vi "SLSC Dynamic Channel Lookups.vi"(6 "SLSCChannelPath":string="SLSCChannelPath", 8 "error in (no error)":errorcluster, 11 "Child Refs":T1[](array[typedef]) format="%.0x") -> (0 "error out":errorcluster, 3 "SLSC Dynamic Inputs":T2[](array[typedef]))   [LabVIEW 2017, in "SLSC EDS System Explorer.lvlib"]
uses:
  SLSC EDS System Explorer.lvlib
  SLSC CD API/SLSC CD Engine/SLSC Dynamic Channel.ctl
  SLSC CD API/SLSC CD Engine/SLSC Datatype.ctl
  <vilib>/NI Veristand/Custom Device API/Custom Device Item Ref.ctl
  <vilib>/NI Veristand/Custom Device API/Get Item Property (String).vi
  <vilib>/NI VeriStand/Custom Device API/Custom Device API.lvlib
  <vilib>/regexp/Match Regular Expression.xnode
  SLSC CD API/SLSC CD Shared/SLSC CD Shared.lvlib
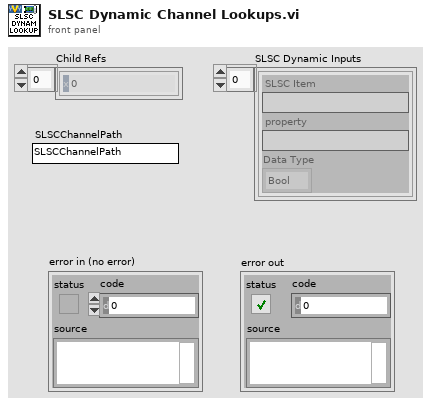
[diagram p1: front panel]
types:
  T1 = typedef "Custom Device API.lvlib/Custom Device Item Ref.ctl" = u64
  T2 = typedef "SLSC CD Shared.lvlib/SLSC Dynamic Channel.ctl" = cluster{"SLSC Item":string, "property":string, "Data Type":T3}
  T3 = typedef "SLSC CD Shared.lvlib/SLSC Datatype.ctl" = enum16{"Bool", "Double", "I32", "I64", "String", "U32", "U64"}
  T4 = enum16{"Bool", "Double", "I32", "I64", "String", "U32", "U64"}
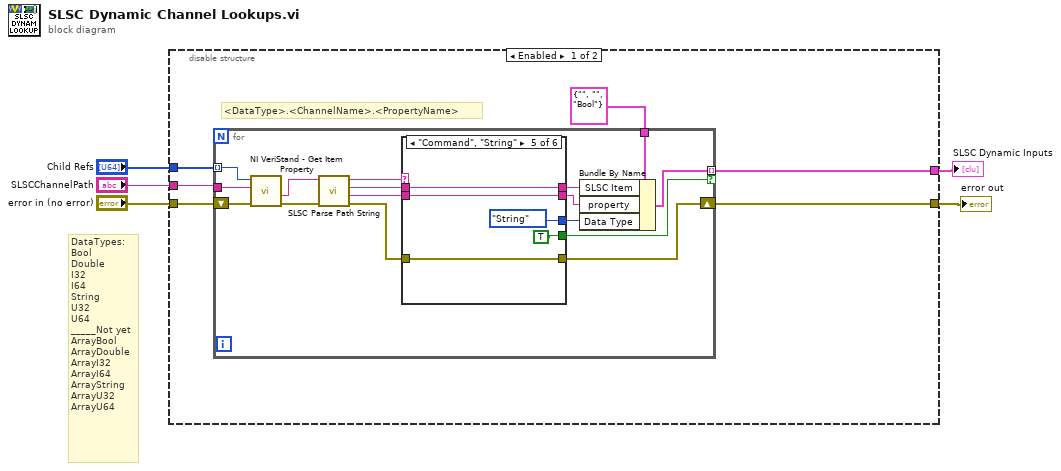
[diagram p0: block diagram]
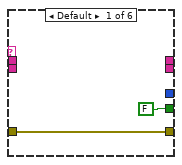
[diagram p2: hidden frame]
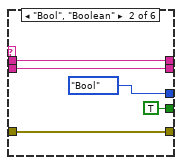
[diagram p3: hidden frame]
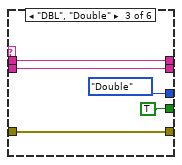
[diagram p4: hidden frame]
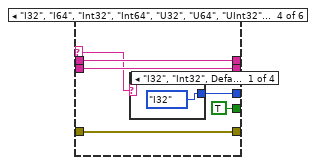
[diagram p5: hidden frame]
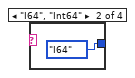
[diagram p6: hidden frame]
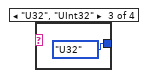
[diagram p7: hidden frame]
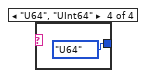
[diagram p8: hidden frame]
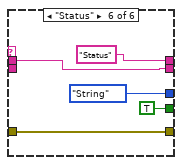
[diagram p9: hidden frame]
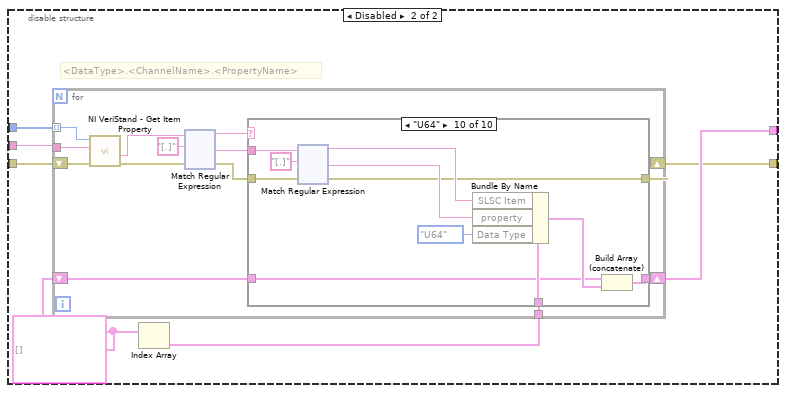
[diagram p10: hidden frame]
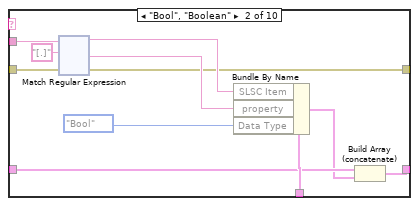
[diagram p12: hidden frame]
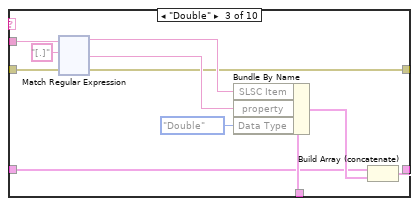
[diagram p13: hidden frame]
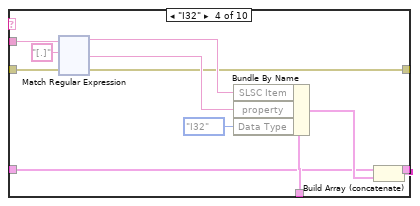
[diagram p14: hidden frame]
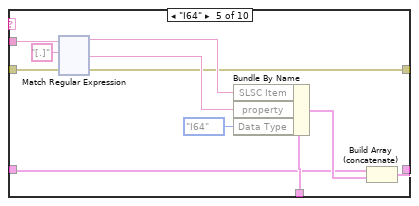
[diagram p15: hidden frame]
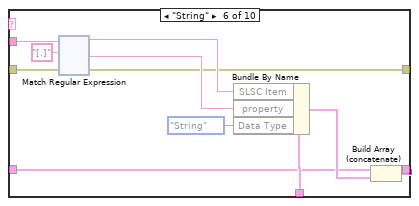
[diagram p16: hidden frame]
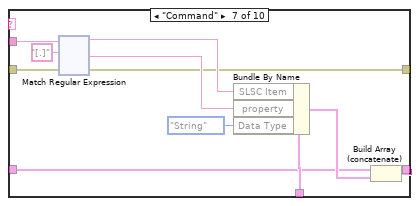
[diagram p17: hidden frame]
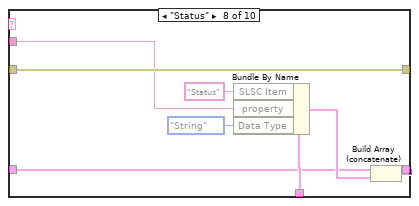
[diagram p18: hidden frame]
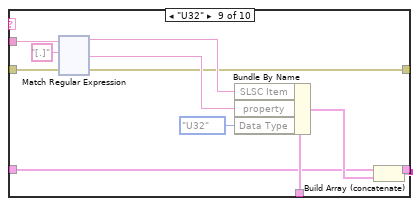
[diagram p19: hidden frame]
diagram:
  # "DataTypes:\nBool\nDouble\nI32\nI64\nString\nU32\nU64\n_____Not yet\nArrayBool\nArrayDouble\nArrayI32\nArrayI64\nArrayString\nArrayU32\nArrayU64"
  n1 = disable-structure shown="Enabled" {
    disable-tunnel: "Child Refs" -> [w11 w66]
    disable-tunnel: "error in (no error)" -> [w10 w65]
    disable-tunnel: [w7 w64] -> w3
    disable-tunnel: [w9 w63] -> w2
    disable-tunnel: "SLSCChannelPath" -> [w8 w62]
    frame Enabled {
      # "<DataType>.<ChannelName>.<PropertyName>"
      n2 = for {
        tunnel: w11 -> [w27] mode=indexing
        tunnel: w8 -> [w26]
        shift-right: [w24] -> w9
        shift-left: w10 -> [w25]
        tunnel: [w21] -> w7 mode=indexing if=w13
        tunnel: T2 {"SLSC Item"="", "property"="", "Data Type"=enum."Bool"} ("SLSC Dynamic Channel") -> [w12]
        n3 = call-poly <vilib>:"NI VeriStand - Get Item Property.vi"("error in (no error)"=w25, "Property Name"=w26, "Item Ref in"=w27) -> ("error out"=w15:errorcluster, "Value"=w23:string)  [unwired: 5 in, 2 out]
        n4 = call "SLSC Parse Path String.vi"("error in (no error)"=w15, "SLSC Channel Path"=w23) -> ("error out"=w14:errorcluster, "Property or Command"=w17:string, "Physical Channel"=w19:string, "Datatype"=w22:string)  [unwired: 6 in]
        n5 = case shown="\"Command\", \"String\"" w22 {
          selector: w22 -> [_ _ _ w41 _ _]
          tunnel: w14 -> [w29 w31 w36 w43 w51 w58]
          tunnel: [w29 w31 w36 w43 w51 w58] -> w24
          tunnel: [_ w34 w39 w45 w54 "Status" ("Physical Channel")] -> w20
          tunnel: w19 -> [_ w34 w39 w45 w54 w55]
          tunnel: [_ w33 w38 w44 w53 w55] -> w18
          tunnel: w17 -> [_ w33 w38 w44 w53 _]
          tunnel: [_ SLSC_Datatype."Bool" ("Data Type") SLSC_Datatype."Double" ("Data Type") w40 SLSC_Datatype."String" ("Data Type") SLSC_Datatype."String" ("Data Type")] -> w16
          tunnel: [FALSE TRUE TRUE TRUE TRUE TRUE] -> w13
          frame Default {
          }
          frame "Bool", "Boolean" {
          }
          frame "DBL", "Double" {
          }
          frame "I32", "I64", "Int32", "Int64", "U32", "U64", "UInt32", "UInt64" {
            n6 = case shown="\"I32\", \"Int32\", Default" w41 {
              tunnel: [SLSC_Datatype."I32" ("Data Type") SLSC_Datatype."I64" ("Data Type") SLSC_Datatype."U32" ("Data Type") SLSC_Datatype."U64" ("Data Type")] -> w40
              frame "I32", "Int32", Default {
              }
              frame "I64", "Int64" {
              }
              frame "U32", "UInt32" {
              }
              frame "U64", "UInt64" {
              }
            }
          }
          frame "Command", "String" {
          }
          frame "Status" {
          }
        }
        n7 = Bundle By Name(cluster=w12, "SLSC Item"=w20, "property"=w18, "Data Type"=w16) -> (w21:T2)
      }
    }
    frame Disabled {
      w60 = T2[] [] ("SLSC Dynamic Inputs")
      # "<DataType>.<ChannelName>.<PropertyName>"
      n8 = Index Array(array=w60) -> (element=w61:T2)  [unwired: 1 in]
      n9 = for {
        tunnel: w66 -> [w79] mode=indexing
        tunnel: w62 -> [w78]
        shift-right: [w67] -> w63
        shift-left: w65 -> [w73]
        tunnel: w61 -> [w70]
        shift-right: [w68] -> w64
        shift-left: w60 -> [w69]
        n10 = call-poly <vilib>:"NI VeriStand - Get Item Property.vi"("error in (no error)"=w73, "Property Name"=w78, "Item Ref in"=w79) -> ("error out"=w71:errorcluster, "Value"=w72:string)  [unwired: 5 in, 2 out]
        n11 = xnode "Match Regular Expression"("input string"=w72, "regular expression"="[.]", "error in"=w71) -> ("before match"=w75:string, "after match"=w76:string, "error out"=w77:errorcluster)  [unwired: 3 in, 2 out]
        n12 = case shown="\"U64\"" w75 {
          tunnel: w76 -> [_ w91 w216 w341 w466 w591 w716 w833 w849 w974]
          tunnel: w77 -> [w81 w90 w215 w340 w465 w590 w715 w834 w848 w973]
          tunnel: w70 -> [_ w87 w210 w337 w462 w587 w712 w839 w845 w970]
          tunnel: w69 -> [w80 w86 w208 w334 w458 w584 w709 w836 w841 w966]
          tunnel: [w80 w85 w211 w333 w459 w583 w708 w835 w843 w967] -> w68
          tunnel: [w81 w83 w207 w332 w457 w582 w707 w834 w840 w965] -> w67
          frame Default {
          }
          frame "Bool", "Boolean" {
            n13 = xnode "Match Regular Expression"("input string"=w91, "regular expression"="[.]", "error in"=w90) -> ("before match"=w89:string, "after match"=w88:string, "error out"=w83:errorcluster)  [unwired: 3 in, 2 out]
            n14 = Bundle By Name(cluster=w87, "SLSC Item"=w89, "property"=w88, "Data Type"=SLSC_Datatype."Bool") -> (w84:T2)
            n15 = Build Array (concatenate)(w86, w84) -> (w85:T2[])
          }
          frame "Double" {
            n16 = xnode "Match Regular Expression"("input string"=w216, "regular expression"="[.]", "error in"=w215) -> ("before match"=w214:string, "after match"=w213:string, "error out"=w207:errorcluster)  [unwired: 3 in, 2 out]
            n17 = Bundle By Name(cluster=w210, "SLSC Item"=w214, "property"=w213, "Data Type"=T4."Double") -> (w209:T2)
            n18 = Build Array (concatenate)(w208, w209) -> (w211:T2[])
          }
          frame "I32" {
            n19 = xnode "Match Regular Expression"("input string"=w341, "regular expression"="[.]", "error in"=w340) -> ("before match"=w339:string, "after match"=w338:string, "error out"=w332:errorcluster)  [unwired: 3 in, 2 out]
            n20 = Bundle By Name(cluster=w337, "SLSC Item"=w339, "property"=w338, "Data Type"=T4."I32") -> (w335:T2)
            n21 = Build Array (concatenate)(w334, w335) -> (w333:T2[])
          }
          frame "I64" {
            n22 = xnode "Match Regular Expression"("input string"=w466, "regular expression"="[.]", "error in"=w465) -> ("before match"=w464:string, "after match"=w463:string, "error out"=w457:errorcluster)  [unwired: 3 in, 2 out]
            n23 = Bundle By Name(cluster=w462, "SLSC Item"=w464, "property"=w463, "Data Type"=T4."I64") -> (w460:T2)
            n24 = Build Array (concatenate)(w458, w460) -> (w459:T2[])
          }
          frame "String" {
            n25 = xnode "Match Regular Expression"("input string"=w591, "regular expression"="[.]", "error in"=w590) -> ("before match"=w589:string, "after match"=w588:string, "error out"=w582:errorcluster)  [unwired: 3 in, 2 out]
            n26 = Bundle By Name(cluster=w587, "SLSC Item"=w589, "property"=w588, "Data Type"=T4."String") -> (w585:T2)
            n27 = Build Array (concatenate)(w584, w585) -> (w583:T2[])
          }
          frame "Command" {
            n28 = xnode "Match Regular Expression"("input string"=w716, "regular expression"="[.]", "error in"=w715) -> ("before match"=w714:string, "after match"=w713:string, "error out"=w707:errorcluster)  [unwired: 3 in, 2 out]
            n29 = Bundle By Name(cluster=w712, "SLSC Item"=w714, "property"=w713, "Data Type"=T4."String") -> (w710:T2)
            n30 = Build Array (concatenate)(w709, w710) -> (w708:T2[])
          }
          frame "Status" {
            n31 = Bundle By Name(cluster=w839, "SLSC Item"="Status", "property"=w833, "Data Type"=T4."String") -> (w837:T2)
            n32 = Build Array (concatenate)(w836, w837) -> (w835:T2[])
          }
          frame "U32" {
            n33 = xnode "Match Regular Expression"("input string"=w849, "regular expression"="[.]", "error in"=w848) -> ("before match"=w847:string, "after match"=w846:string, "error out"=w840:errorcluster)  [unwired: 3 in, 2 out]
            n34 = Bundle By Name(cluster=w845, "SLSC Item"=w847, "property"=w846, "Data Type"=T4."U32") -> (w842:T2)
            n35 = Build Array (concatenate)(w841, w842) -> (w843:T2[])
          }
          frame "U64" {
            n36 = xnode "Match Regular Expression"("input string"=w974, "regular expression"="[.]", "error in"=w973) -> ("before match"=w972:string, "after match"=w971:string, "error out"=w965:errorcluster)  [unwired: 3 in, 2 out]
            n37 = Bundle By Name(cluster=w970, "SLSC Item"=w972, "property"=w971, "Data Type"=T4."U64") -> (w968:T2)
            n38 = Build Array (concatenate)(w966, w968) -> (w967:T2[])
          }
        }
      }
    }
  }
  "SLSC Dynamic Inputs" <- w3
  "error out" <- w2
